vi "GSI-HVSwitch2.write data.vi"(0 "i ref in":refnum<vi>, 1 "SetVoltage SW0":dbl, 2 "SetVoltage SW1":dbl, 3 "ms timeout (10000)":i32=10000, 5 "error in (no error)":errorcluster) -> (14 "i ref out":refnum<vi>, 17 "timed out":bool, 19 "error out":errorcluster)   [LabVIEW 2014, in "GSI-HVSwitch2.lvlib"]
doc: "Writes the data to the instrument."
uses:
  GSI-HVSwitch2.lvlib
  CSCore/CSSystem/CoreDefs/CoreDefs.error_type.ctl
  CSCore/CSSystem/CoreLib/CoreLib.lvlib
  CSCore/CSApplicationBaseClasses/DeviceBase/DeviceBase.lvlib
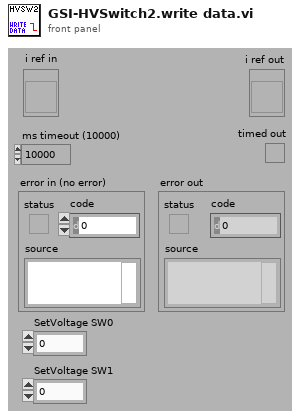
[diagram p1: front panel]
types:
  T1 = typedef "CoreDefs.error_type.ctl" = enum16{"no error", "can't load process", "can't unload process", "process does not exist", "can't install process", "can't remove process", "unknown function", "time out", "can't execute function", "duplicate queue name", "super not found", "caller queue invalid", "can't ping process", "unknown error", "VISA Error", "VISA timeout", "GPIB timeout", "GPIB error", "communication error", "data type mismatch", "can't read data from OPC server", "can't write data to OPC server", "OET error", "function not implemented", "process already exists", "invalid Shared Variable name", "error writing Shared Variable", "error reading Shared Variable", "invalid client name", "corrupt database", "unknown class", "call not authorized", "parameter out of range", "OET timeout: can't get data to modify", "invalid queue name", "requested operation incompatible with current state", "event undefined", "event disabled", "state undefined", "caller is not a friend", "EventBuilder: bad eventID", "EventBuilder: no DAQ devices", "a thread must not stop itself", "UNUSED ELEMENT4", "DiscArchiver: eventData incomplete", "DiscArchiver: eventData does not belong to run", "DiscArchiver: can't open file", "DiscArchiver: can't write to file", "DiscArchiver: available disc space low", "can't acquire semaphore", "error reading data from database", "notifier object is not existing", "can't register process", "can't unregister process", "illegal event type", "object disabled", "object already exists", "can't change state", "Instrument not found", "no connection to remote node", "invalid reference", "N/A", "UNUSED ELEMENT 1", "element not found", "illegal TCP/IP connection detected", "object does not exist", "invalid access ID", "unknown CS system", "invalid privilige", "unsupported data type", "unsupported server type", "IO server already exists", "Shared Variable already exists"}
  T2 = typedef "GSI-HVSwitch2.lvlib/GSI-HVSwitch2.i attribute.ctl" = cluster{"SDEX VISA Cluster":T3, "SetVoltage SW0":dbl, "SetVoltage SW1":dbl, "ActTempAmp":dbl, "ActTempPS1":dbl, "ActTempPS2":dbl, "mode":T6, "interfaceInitialized":bool, "serviceIDs":cluster{"nomVoltage0ID":i32, "nomVoltage1ID":i32, "actTempAmpID":i32, "actTempPS1ID":i32, "actTempPS2ID":i32, "modeID":i32}, "usedChannels":i32}
  T3 = typedef "SDEXDriver.lvlib/SDEX.VISA Control.ctl" = cluster{"VISA resource name":refnum<visa-resource-name>, "HEX address":u16, "VISA Timeout Value (1000 ms)":u32, "Lock Timeout (1000 ms)":u32, "semaphore":T4, "Baud rate":u32, "revision":T5, "deviceInfo":string}
  T4 = typedef "Semaphore RefNum" = refnum<k1>
  T5 = typedef "SDEXDriver.lvlib/SDEX.revisionType.ctl" = enum16{"unknown", "hvamp3", "hvswi1", "htrp0", "WDG0"}
  T6 = typedef "GSI-HVSwitch2.lvlib/GSI-HVSwitch2.mode.ctl" = enum16{"unknown", "switch", "stepper"}
  T7 = typedef "DeviceBase.lvlib/DeviceBase.i attribute.ctl" = cluster{"deviceState":i32, "deviceStateID":i32, "deviceID":string, "deviceIDID":i32, "advancedGUIClass":string, "advancedGUIClassID":i32}
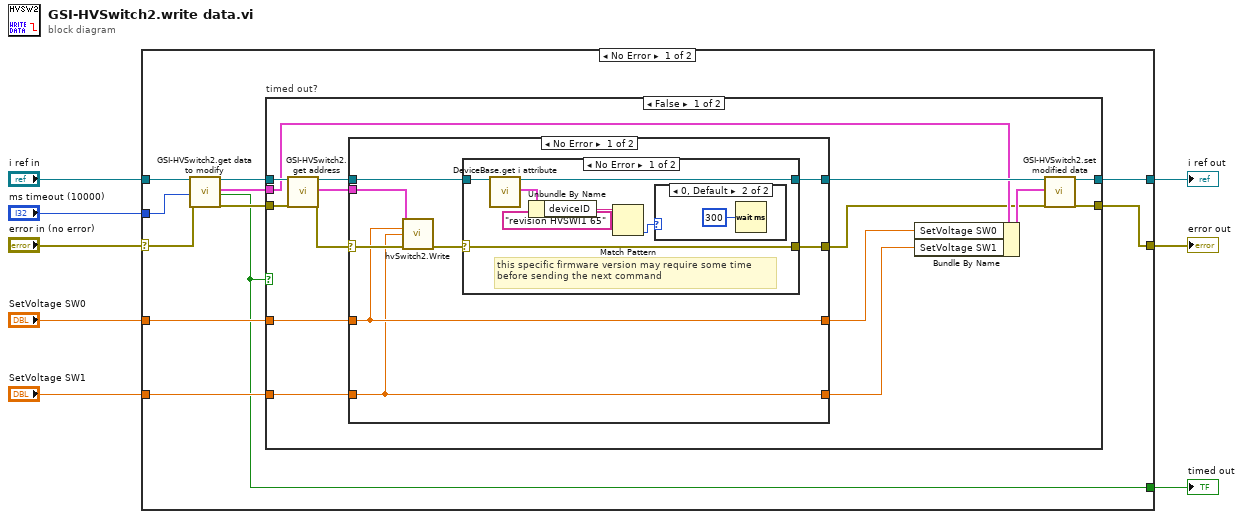
[diagram p0: block diagram]
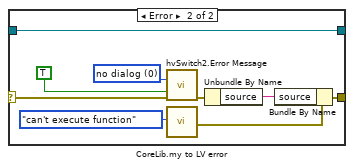
[diagram p3: hidden frame]
diagram:
  n1 = case shown="No Error" "error in (no error)" {
    selector: "error in (no error)" -> [w9 w66]
    tunnel: [w19 w66] -> w8
    tunnel: [w18 w67] -> w7
    tunnel: "SetVoltage SW0" -> [w17 _]
    tunnel: "SetVoltage SW1" -> [w16 _]
    tunnel: "i ref in" -> [w15 w67]
    tunnel: "ms timeout (10000)" -> [w14 _]
    tunnel: [w12 _] -> w2
    frame No Error {
      n2 = call "GSI-HVSwitch2.get data to modify.vi"("i ref in"=w15, "ms timeout (10000)"=w14, "error in (no error)"=w9) -> ("i ref out"=w11:refnum<vi>, "i attribute"=w10:T2, "timed out"=w12:bool, "error out"=w13:errorcluster)  [unwired: 13 in]
      n3 = case "timed out?" shown="False" w12 {
        tunnel: [w26 w64] -> w19
        tunnel: [w27 w65] -> w18
        tunnel: w17 -> [w31 _]
        tunnel: w16 -> [w30 _]
        tunnel: w13 -> [w29 w64]
        tunnel: w11 -> [w28 w65]
        tunnel: w10 -> [w24 _]
        frame False {
          n4 = call "GSI-HVSwitch2.get address.vi"("i ref in"=w28, "error in (no error)"=w29) -> ("i ref out"=w32:refnum<vi>, "SDEX address"=w34:T3, "error out"=w33:errorcluster)  [unwired: 15 in]
          n5 = case shown="No Error" w33 {
            selector: w33 -> [w42 w63]
            tunnel: w34 -> [w41 _]
            tunnel: [w37 w63] -> w22
            tunnel: [w35 w62] -> w25
            tunnel: w32 -> [w36 w62]
            tunnel: w31 -> [w40 w61]
            tunnel: w30 -> [w39 w60]
            tunnel: [w40 w61] -> w21
            tunnel: [w39 w60] -> w20
            frame No Error {
              n6 = call "hvSwitch2.Write.vi"("SDEX VISA Cluster"=w41, "SetVoltage SW0"=w40, "SetVoltage SW1"=w39, "error in (no error)"=w42) -> ("error out"=w38:errorcluster)  [unwired: 10 in, 1 out]
              n7 = case shown="No Error" w38 {
                selector: w38 -> [w49 w57]
                tunnel: [w49 w55] -> w37
                tunnel: w36 -> [w48 w51]
                tunnel: [w47 w51] -> w35
                frame No Error {
                  # "this specific firmware version may require some time\nbefore sending the next command"
                  n8 = call "DeviceBase.get i attribute.vi"("i ref in"=w48) -> ("i ref out"=w47:refnum<vi>, "i attribute"=w46:T7)  [unwired: 16 in, 1 out]
                  n9 = Unbundle By Name(w46) -> ("deviceID"=w45:string)
                  n10 = Match Pattern(string=w45, regular expression="revision HVSWI1 65") -> (offset past match=w43:i32)  [unwired: 1 in, 3 out]
                  n11 = case shown="0, Default" w43 {
                    frame -1 {
                    }
                    frame 0, Default {
                      n12 = Wait (ms)(milliseconds to wait=u32 300) -> ()  [unwired: 1 out]
                    }
                  }
                }
                frame Error {
                  w59 = u16 0 items=["no dialog", "OK message", "continue or stop message"] ("type of dialog (no dialog: 0)")
                  n13 = call "hvSwitch2.Error Message.vi"("Type of Dialog (0: No Dialog)"=w59, "append msg 2 src"=TRUE ("add message to source"), "error in (no error)"=w57) -> ("error out"=w53:errorcluster)  [unwired: 8 in, 4 out]
                  n14 = call "CoreLib.my to LV error.vi"("ErrorTypes"=CoreDefs.error_type."can't execute function") -> ("myErrorCluster"=w54:errorcluster)  [unwired: 17 in, 1 out]
                  n15 = Unbundle By Name(w53) -> ("source"=w52:string)
                  n16 = Bundle By Name(cluster=w54, "source"=w52) -> (w55:errorcluster)
                }
              }
            }
            frame Error {
            }
          }
          n17 = Bundle By Name(cluster=w24, "SetVoltage SW0"=w21, "SetVoltage SW1"=w20) -> (w23:T2)
          n18 = call "GSI-HVSwitch2.set modified data.vi"("i ref in"=w25, "i attribute"=w23, "error in (no error)"=w22) -> ("i ref out"=w27:refnum<vi>, "error out"=w26:errorcluster)  [unwired: 15 in]
        }
        frame True {
        }
      }
    }
    frame Error {
    }
  }
  "error out" <- w8
  "i ref out" <- w7
  "timed out" <- w2
